vi "Radau5_Implicit RK Manager.vi"(9 "Jac Variant":variant, 10 "Jac Refnum":refnum<vi>, 11 "Simulation Data In":T1 {"Absolute tolerance" format="%.1e"; "Relative tolerance" format="%.1e"; "Output of T" format="%.1e"; "proposed step size" format="%.1e"; "min step size" format="%.1e"; "max step size" format="%.1e"; "final time" format="%.1e"; "step size" format="%.1e"; "initial time" format="%.1e"}) -> (3 "Simulation Data Out":T1 {"Absolute tolerance" format="%.1e"; "Relative tolerance" format="%.1e"; "Output of T" format="%.1e"; "proposed step size" format="%.1e"; "min step size" format="%.1e"; "max step size" format="%.1e"; "final time" format="%.1e"; "step size" format="%.1e"; "initial time" format="%.1e"})   [LabVIEW 2017, in "NI_DAE.lvlib"]
uses:
  <vilib>/gmath/NI_DAE.lvlib
  <vilib>/gmath/dae.llb/Radau5_Simulation Data.ctl
  <vilib>/gmath/dae.llb/Radau5_Diag Eval Stage.ctl
  <vilib>/gmath/dae.llb/Radau5_RK Status.ctl
  <vilib>/Analysis/baseanly.llb/A x Vector (Optimized).vi
  <vilib>/gmath/NI_Gmath.lvlib
  <vilib>/Analysis/NI_AALBase.lvlib
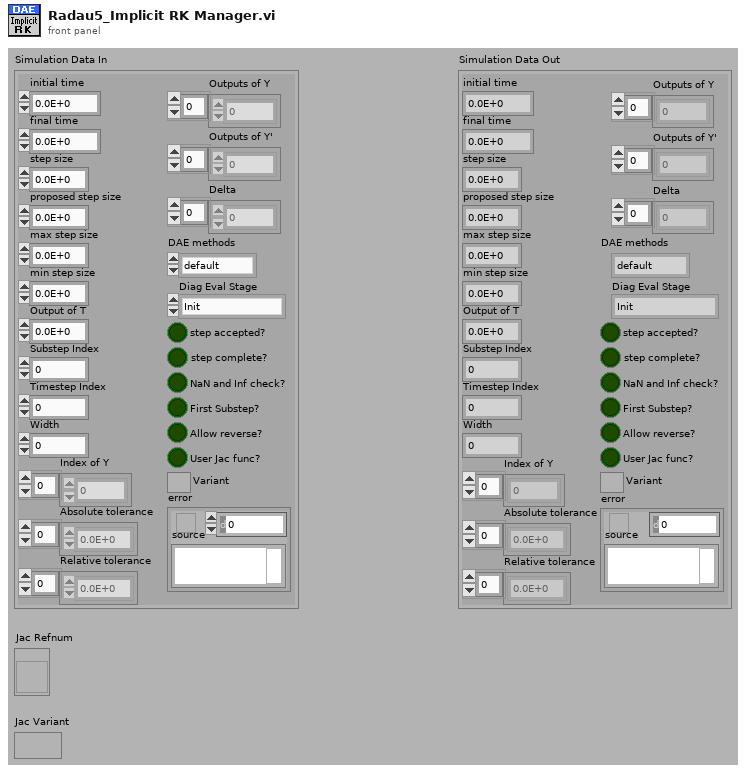
[diagram p1: front panel]
types:
  T1 = typedef "NI_DAE.lvlib/Radau5_Simulation Data.ctl" = cluster{"initial time":dbl, "final time":dbl, "step size":dbl, "proposed step size":dbl, "max step size":dbl, "min step size":dbl, "Output of T":dbl, "Substep Index":i32, "Timestep Index":i32, "Width":i32, "Absolute tolerance":dbl[], "Relative tolerance":dbl[], "Outputs of Y":dbl[], "Outputs of Y'":dbl[], "Delta":dbl[], "DAE methods":enum16{"default", "Radau IIA"}, "Diag Eval Stage":T2, "step accepted?":bool, "step complete?":bool, "NaN and Inf check?":bool, "First Substep?":bool, "Allow reverse?":bool, "error":errorcluster, "User Jac func?":bool, "Variant":variant, "Index of Y":i8[]}
  T2 = typedef "NI_DAE.lvlib/Radau5_Diag Eval Stage.ctl" = enum16{"Init", "Running", "Final", "End"}
  T3 = typedef "NI_DAE.lvlib/Radau5_RK Status.ctl" = enum16{"Init", "Predict", "Jacobian", "Newton", "error eval y y'", "error eval calc", "next step updata", "reset RK"}
  T4 = typedef "NI_DAE.lvlib/Radau5_Implicit RK Data.ctl" = cluster{"time":dbl, "Old time":dbl, "Step size":dbl, "Old step size":dbl, "Width":i32, "Newton index":i32, "Old Y(k)":dbl[], "Old Y'":dbl[], "Stage time":dbl[], "Old stage time":dbl[], "Increment Z":dbl[], "Delta Z":dbl[], "U":dbl[], "Old Delta Z":dbl[], "Y(k)":dbl[], "Y'":dbl[], "ErrorTolerance":dbl[], "Local error k+1":dbl[], "Old Local error k":dbl[], "Stage value of Y":dbl[][], "Stage value of Y'":dbl[][], "Old Stage value of Y":dbl[][], "Old Stage value of Y'":dbl[][], "RK status":T3, "do Jac?":bool, "Old Jac?":bool, "Do Newton?":bool, "Matrix J":T5, "Matrix M":T5, "Inverse of JM_1 matrix ":T5, "Inverse of JM_2 matrix":T6}
  T5 = typedef "NI_Matrix.lvlib/RealMatrix.ctl" = dbl[][]
  T6 = typedef "NI_Matrix.lvlib/ComplexMatrix.ctl" = cdb[][]
  T7 = typedef "NI_DAE.lvlib/Radau5_Newton Status.ctl" = enum16{"success", "unsuccess(iteration diverge)", "unsuccess(exceed max_N)", "unsuccess(conv rate too slow)", "Continue next Newton"}
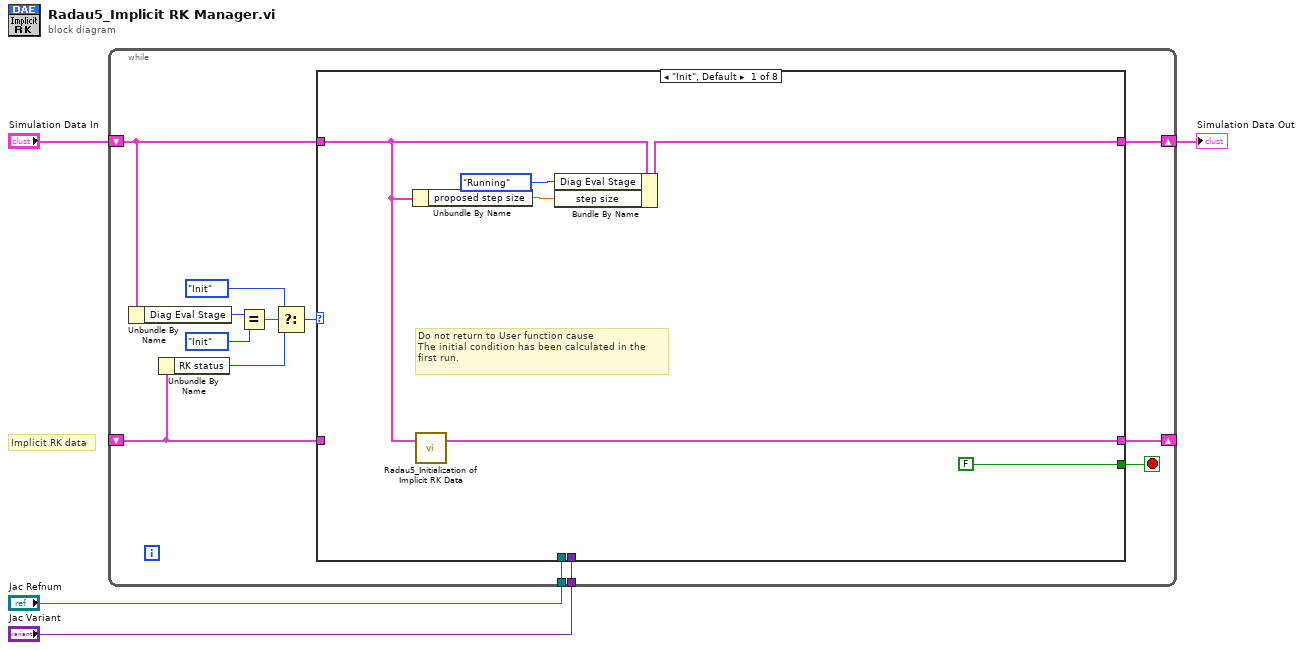
[diagram p0: block diagram]
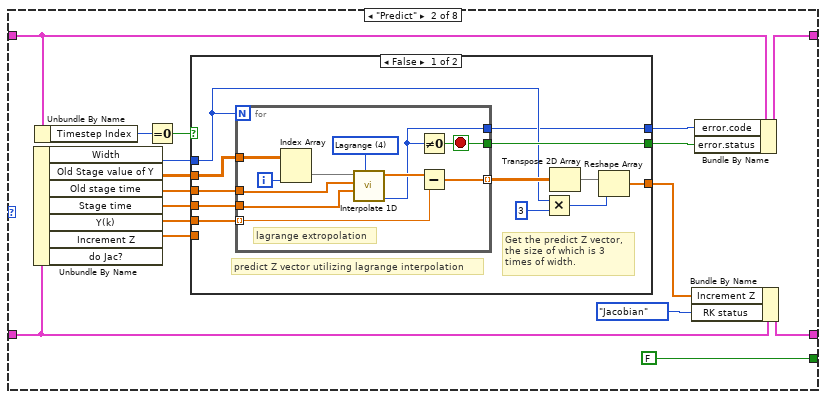
[diagram p2: hidden frame]
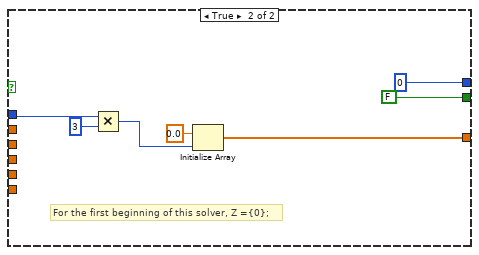
[diagram p3: hidden frame]
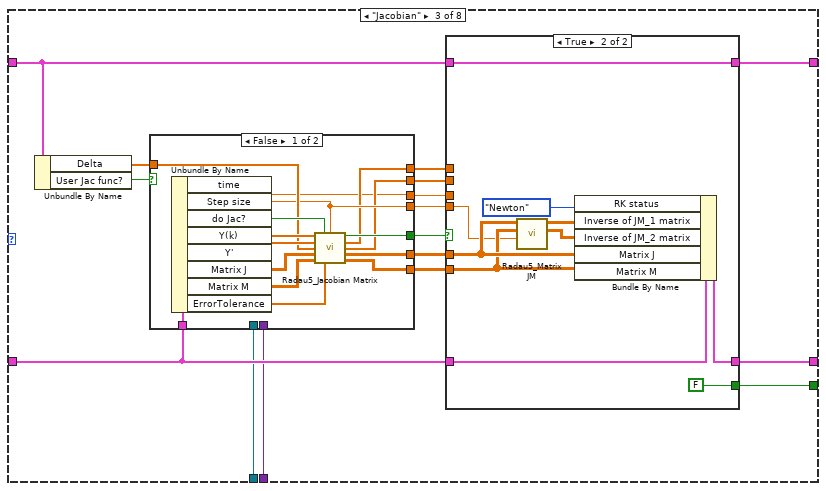
[diagram p4: hidden frame]
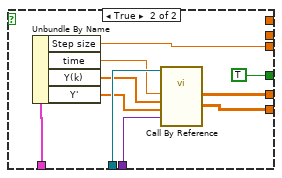
[diagram p5: hidden frame]
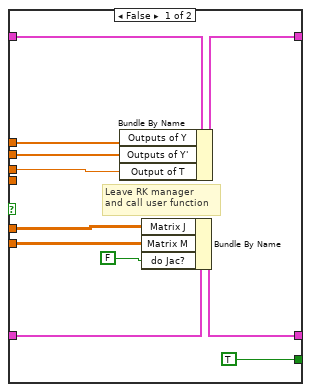
[diagram p6: hidden frame]
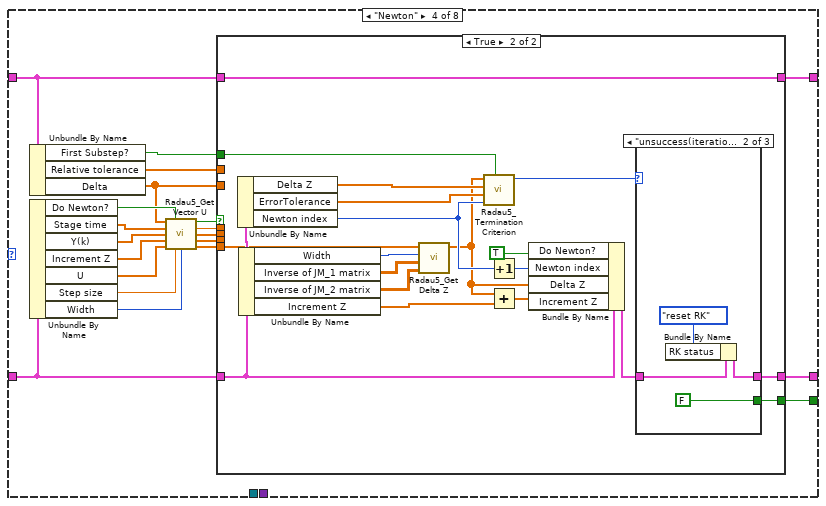
[diagram p7: hidden frame]
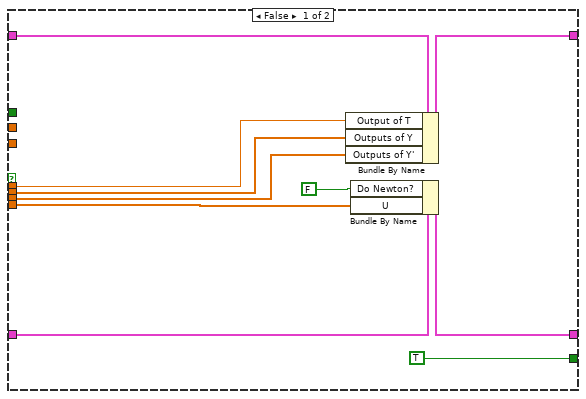
[diagram p8: hidden frame]
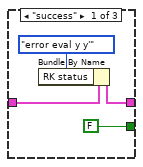
[diagram p9: hidden frame]
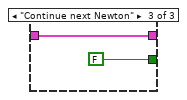
[diagram p10: hidden frame]
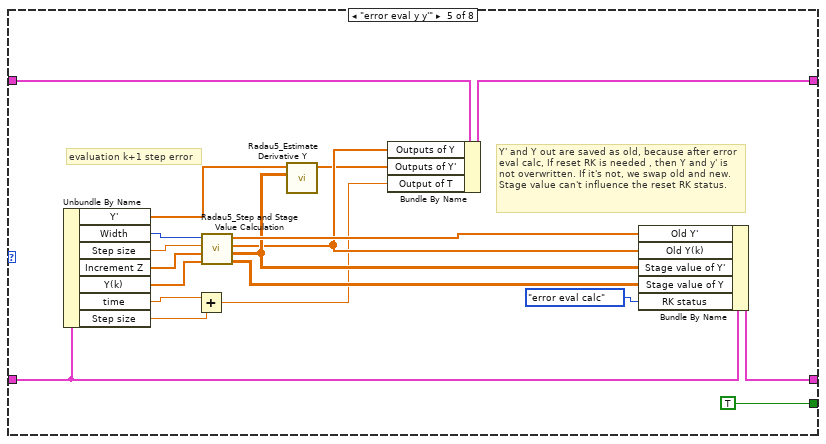
[diagram p11: hidden frame]
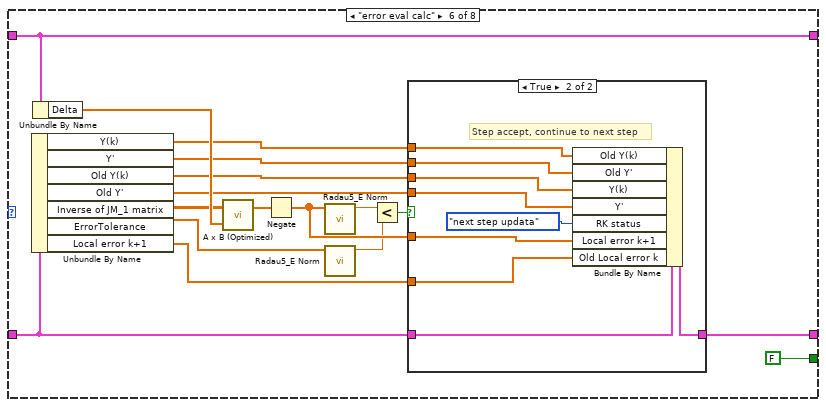
[diagram p12: hidden frame]
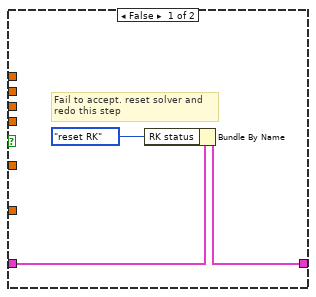
[diagram p13: hidden frame]
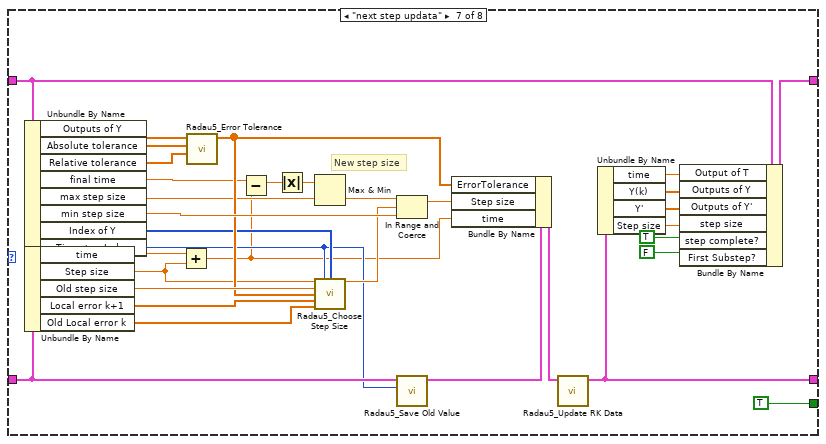
[diagram p14: hidden frame]
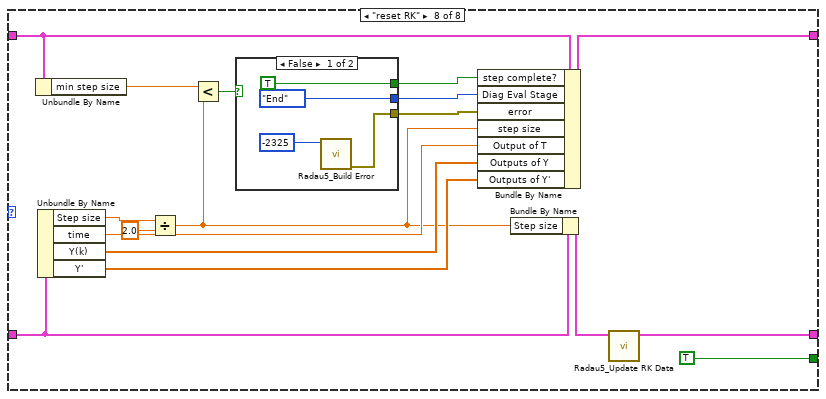
[diagram p15: hidden frame]
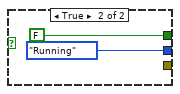
[diagram p16: hidden frame]
diagram:
  # "Implicit RK data"
  n1 = while {
    shift-right: [w7] -> _
    shift-left: _ -> [w8]
    shift-right: [w9] -> w3
    shift-left: "Simulation Data In" -> [w10]
    tunnel: "Jac Refnum" -> [w6]
    tunnel: "Jac Variant" -> [w5]
    stop <- w17 stop-if-true
    n2 = Unbundle By Name(w10) -> ("Diag Eval Stage"=w16:T2)
    n3 = Unbundle By Name(w8) -> ("RK status"=w12:T3)
    n4 = Equal?(x=w16, y=Radau5_Diag_Eval_Stage."Init") -> (x = y?=w14:bool)
    n5 = Select(t=Radau5_RK_Status."Init" ("RK status"), s=w14, f=w12) -> (s? t:f=w11:T3)
    n6 = case shown="\"Init\", Default" w11 {
      tunnel: w8 -> [_ w29 w84 w146 w207 w226 w266 w275]
      tunnel: [w22 w39 w81 w144 w205 w224 w260 w276] -> w7
      tunnel: [FALSE FALSE w79 w142 TRUE ("Newton flag") FALSE ("Newton flag") TRUE ("Newton flag") TRUE ("Newton flag")] -> w17
      tunnel: w10 -> [w19 w38 w78 w145 w210 w223 w262 w287]
      tunnel: [w20 w37 w75 w141 w209 w223 w261 w278] -> w9
      tunnel: w6 -> [_ _ w73 _ _ _ _ _]
      tunnel: w5 -> [_ _ w71 _ _ _ _ _]
      frame "Init", Default {
        # "Do not return to User function cause\nThe initial condition has been calculated in the \nfirst run."
        n7 = Unbundle By Name(w19) -> ("proposed step size"=w18:dbl)
        n8 = call <vilib>:"Radau5_Initialization of Implicit RK Data.vi"("Simulation Data"=w19) -> ("Implicit RK Data"=w22:T4)  [unwired: 2 in]
        n9 = Bundle By Name(cluster=w19, "Diag Eval Stage"=Radau5_Diag_Eval_Stage."Running", "step size"=w18) -> (w20:T1)
      }
      frame "Predict" {
        n10 = Unbundle By Name(w29) -> ("Width"=w34:i32, "Old Stage value of Y"=w33:dbl[][], "Old stage time"=w32:dbl[], "Stage time"=w31:dbl[], "Y(k)"=w30:dbl[], "Increment Z"=w28:dbl[])  [unwired: 1 out]
        n11 = Unbundle By Name(w38) -> ("Timestep Index"=w25:i32)
        n12 = Equal To 0?(x=w25) -> (x = 0?=w26:bool)
        n13 = case shown="False" w26 {
          tunnel: [w48 FALSE] -> w36
          tunnel: [w41 0 ("error")] -> w35
          tunnel: w34 -> [w47 w66]
          tunnel: w33 -> [w46 _]
          tunnel: w32 -> [w45 _]
          tunnel: w31 -> [w44 _]
          tunnel: w30 -> [w43 _]
          tunnel: [w42 w67] -> w27
          tunnel: w28 -> [_ _]
          frame False {
            # "Get the predict Z vector, \nthe size of which is 3 times of width."
            # "predict Z vector utilizing lagrange interpolation"
            n14 = for {
              N: w47 -> [_]
              tunnel: w45 -> [w59]
              tunnel: w46 -> [w62]
              tunnel: w44 -> [w58]
              tunnel: w43 -> [w56] mode=indexing
              tunnel: [w55] -> w52 mode=indexing
              tunnel: [w54] -> w48
              tunnel: [w53] -> w41
              i -> [w61]
              stop <- w54 stop-if-true
              w63 = 4 items=["nearest", "linear", "spline", "cubic Hermite", "Lagrange"] ("method")
              # "lagrange extropolation"
              n15 = Index Array(array=w62, index (col)=w61) -> (element=w60:dbl[])  [unwired: 1 in]
              n16 = call <vilib>:"Interpolate 1D.vi"("method"=w63, "xi"=w58, "X"=w59, "Y"=w60) -> ("error"=w53:i32, "yi"=w57:dbl[])  [unwired: 2 in, 4 out]
              n17 = Not Equal To 0?(x=w53) -> (x != 0?=w54:bool)
              n18 = Subtract(x=w57, y=w56) -> (x-y=w55:dbl[])
            }
            n19 = Multiply(x=w47, y=3 ("x")) -> (x*y=w49:i32)
            n20 = Transpose 2D Array(2D array=w52) -> (transposed array=w51:dbl[][])
            n21 = Reshape Array(w51, w49) -> (w42:dbl[])
          }
          frame True {
            # "For the first beginning of this solver, Z ={0};"
            n22 = Multiply(x=w66, y=3) -> (x*y=w64:i32)
            n23 = Initialize Array(0.0 ("element"), w64) -> (w67:dbl[])
          }
        }
        n24 = Bundle By Name(cluster=w29, "Increment Z"=w27, "RK status"=Radau5_RK_Status."Jacobian") -> (w39:T4)
        n25 = Bundle By Name(cluster=w38, "error.code"=w35, "error.status"=w36) -> (w37:T1)
      }
      frame "Jacobian" {
        n26 = Unbundle By Name(w78) -> ("Delta"=w86:dbl[], "User Jac func?"=w72:bool)
        n27 = case shown="False" w72 {
          tunnel: w86 -> [w95 _]
          tunnel: [w94 TRUE ("Ready")] -> w85
          tunnel: w84 -> [w93 w111]
          tunnel: [w92 w106] -> w83
          tunnel: [w91 w105] -> w82
          tunnel: [w90 w103] -> w80
          tunnel: [w89 _] -> w77
          tunnel: [w88 _] -> w76
          tunnel: [w87 _] -> w74
          tunnel: w73 -> [_ w110]
          tunnel: w71 -> [_ w102]
          frame False {
            n28 = Unbundle By Name(w93) -> ("time"=w87:dbl, "Step size"=w90:dbl, "do Jac?"=w96:bool, "Y(k)"=w97:dbl[], "Y'"=w98:dbl[], "Matrix J"=w101:T5, "Matrix M"=w100:T5, "ErrorTolerance"=w99:dbl[])
            n29 = call <vilib>:"Radau5_Jacobian Matrix.vi"("Y(k)"=w97, "do Jac?"=w96, "Step size"=w90, "Y'"=w98, "Fout"=w95, "Matrix J"=w101, "Matrix M"=w100, "ErrorTolerance"=w99) -> ("Ready"=w94:bool, "Y(k)"=w89:dbl[], "Y'"=w88:dbl[], "Matrix J"=w92:T5, "Matrix M"=w91:T5)  [unwired: 3 in]
          }
          frame True {
            n30 = Unbundle By Name(w111) -> ("Step size"=w103:dbl, "time"=w109:dbl, "Y(k)"=w108:dbl[], "Y'"=w107:dbl[])
            n31 = call-by-ref "?"(reference=w110, "Variant"=w102, "Y'"=w107, "Y"=w108, "Time"=w109) -> ("Real Matrix 2"=w105:T5, "Real Matrix"=w106:T5)  [unwired: 1 in, 3 out]
          }
        }
        n32 = case shown="True" w85 {
          tunnel: w84 -> [w121 w132]
          tunnel: w83 -> [w120 w130]
          tunnel: w82 -> [w119 w129]
          tunnel: [w118 w131] -> w81
          tunnel: w80 -> [_ w126]
          tunnel: [TRUE FALSE] -> w79
          tunnel: w78 -> [w116 w124]
          tunnel: w77 -> [w115 _]
          tunnel: w76 -> [w114 _]
          tunnel: [w113 w124] -> w75
          tunnel: w74 -> [w112 _]
          frame False {
            # "Leave RK manager\nand call user function"
            n33 = Bundle By Name(cluster=w116, "Outputs of Y"=w115, "Outputs of Y'"=w114, "Output of T"=w112) -> (w113:T1)
            n34 = Bundle By Name(cluster=w121, "Matrix J"=w120, "Matrix M"=w119, "do Jac?"=FALSE) -> (w118:T4)
          }
          frame True {
            n35 = call <vilib>:"Radau5_Matrix JM.vi"("Step size"=w126, "Matrix M"=w129, "Matrix J"=w130) -> ("Inverse of Matrix JM_2"=w127:T6, "Inverse of Matrix JM_1"=w128:T5)  [unwired: 7 in]
            n36 = Bundle By Name(cluster=w132, "RK status"=Radau5_RK_Status."Newton", "Inverse of JM_1 matrix"=w128, "Inverse of JM_2 matrix"=w127, "Matrix J"=w130, "Matrix M"=w129) -> (w131:T4)
          }
        }
      }
      frame "Newton" {
        n37 = Unbundle By Name(w145) -> ("First Substep?"=w134:bool, "Relative tolerance"=w143:dbl[], "Delta"=w135:dbl[])
        n38 = Unbundle By Name(w146) -> ("Do Newton?"=w139:bool, "Stage time"=w136:dbl[], "Y(k)"=w137:dbl[], "Increment Z"=w138:dbl[], "U"=w152:dbl[], "Step size"=w133:dbl, "Width"=w140:i32)
        n39 = call <vilib>:"Radau5_Get Vector U.vi"("Delta In"=w135, "Flag"=w139, "Stage time"=w136, "Step Value Y"=w137, "Vector Z in"=w138, "Vector U in"=w152, "Step size"=w133, "Width"=w140) -> ("Vector U Ready?"=w151:bool, "Stage time out"=w150:dbl, "Stage Y out"=w149:dbl[], "Stage Y' out"=w148:dbl[], "Vector U out"=w147:dbl[])  [unwired: 3 in]
        n40 = case shown="True" w151 {
          tunnel: w150 -> [w160 _]
          tunnel: w149 -> [w155 _]
          tunnel: w148 -> [w154 _]
          tunnel: w147 -> [w156 w171]
          tunnel: w146 -> [w157 w178]
          tunnel: w145 -> [w161 w165]
          tunnel: [w158 w168] -> w144
          tunnel: w135 -> [_ _]
          tunnel: w143 -> [_ _]
          tunnel: [TRUE ("Newton flag") w175] -> w142
          tunnel: [w159 w165] -> w141
          tunnel: w134 -> [_ w167]
          frame False {
            n41 = Bundle By Name(cluster=w161, "Output of T"=w160, "Outputs of Y"=w155, "Outputs of Y'"=w154) -> (w159:T1)
            n42 = Bundle By Name(cluster=w157, "Do Newton?"=FALSE, "U"=w156) -> (w158:T4)
          }
          frame True {
            n43 = Unbundle By Name(w178) -> ("Delta Z"=w164:dbl[], "ErrorTolerance"=w169:dbl[], "Newton index"=w166:i32)
            n44 = Unbundle By Name(w178) -> ("Width"=w172:i32, "Inverse of JM_1 matrix"=w181:T5, "Inverse of JM_2 matrix"=w180:T6, "Increment Z"=w170:dbl[])
            n45 = call <vilib>:"Radau5_Get Delta Z.vi"("Inverse Matrix JM_2"=w180, "Inverse Matrix JM_1"=w181, "Width"=w172, "Vector U in"=w171) -> ("Delta Z out"=w163:dbl[])  [unwired: 7 in]
            n46 = call <vilib>:"Radau5_Termination Criterion.vi"("First call?"=w167, "Newton index"=w166, "Error TOL"=w169, "Old Delta Z"=w164, "Delta Z"=w163) -> ("Newton status"=w177:T7)  [unwired: 6 in]
            n47 = Increment(x=w166) -> (x+1=w174:i32)
            n48 = Add(x=w163, y=w170) -> (x+y=w179:dbl[])
            n49 = Bundle By Name(cluster=w178, "Do Newton?"=TRUE, "Newton index"=w174, "Delta Z"=w163, "Increment Z"=w179) -> (w176:T4)
            n50 = case shown="\"unsuccess(iteration diverge)\", Default" w177 {
              tunnel: w176 -> [w185 w188 w191]
              tunnel: [w183 w187 w191] -> w168
              tunnel: [FALSE ("Newton flag") FALSE ("Newton flag") FALSE ("Newton flag")] -> w175
              frame "success" {
                n51 = Bundle By Name(cluster=w185, "RK status"=Radau5_RK_Status."error eval y y'") -> (w183:T4)
              }
              frame "unsuccess(iteration diverge)", Default {
                n52 = Bundle By Name(cluster=w188, "RK status"=Radau5_RK_Status."reset RK") -> (w187:T4)
              }
              frame "Continue next Newton" {
              }
            }
          }
        }
      }
      frame "error eval y y'" {
        # "Y' and Y out are saved as old, because after error eval calc, If reset RK is needed , then Y and y' is not overwritten. If it's not, we swap old and new.\nStage value can't influence the reset RK status."
        # "evaluation k+1 step error"
        n53 = Unbundle By Name(w207) -> ("Y'"=w194:dbl[], "Width"=w204:i32, "Step size"=w192:dbl, "Increment Z"=w203:dbl[], "Y(k)"=w202:dbl[], "time"=w196:dbl, "Step size"=w197:dbl)
        n54 = Add(x=w196, y=w197) -> (x+y=w195:dbl)
        n55 = call <vilib>:"Radau5_Step and Stage Value Calculation.vi"("Y(k)"=w202, "Increment Z"=w203, "Step size"=w192, "Width"=w204) -> ("Stage value of Y"=w200:dbl[][], "Stage value of Y'"=w199:dbl[][], "Y(k+1) out"=w198:dbl[], "Y'(k+1) out"=w201:dbl[])  [unwired: 4 in]
        n56 = call <vilib>:"Radau5_Estimate Derivative Y.vi"("Stage Y'"=w199, "Old Y'"=w194) -> ("Estimate Y' out"=w193:dbl[])  [unwired: 9 in]
        n57 = Bundle By Name(cluster=w210, "Outputs of Y"=w198, "Outputs of Y'"=w193, "Output of T"=w195) -> (w209:T1)
        n58 = Bundle By Name(cluster=w207, "Old Y'"=w201, "Old Y(k)"=w198, "Stage value of Y'"=w199, "Stage value of Y"=w200, "RK status"=Radau5_RK_Status."error eval calc") -> (w205:T4)
      }
      frame "error eval calc" {
        n59 = Unbundle By Name(w226) -> ("Y(k)"=w219:dbl[], "Y'"=w218:dbl[], "Old Y(k)"=w217:dbl[], "Old Y'"=w216:dbl[], "Inverse of JM_1 matrix"=w220:T5, "ErrorTolerance"=w215:dbl[], "Local error k+1"=w225:dbl[])
        n60 = Unbundle By Name(w223) -> ("Delta"=w227:dbl[])
        n61 = call-poly <vilib>:"A x B (Optimized).vi"("Vector"=w227, "A"=w220) -> ("A x Vector"=w221:dbl[])  [unwired: 1 out]
        n62 = Negate(x=w221) -> (-x=w214:dbl[])
        n63 = call <vilib>:"Radau5_E Norm.vi"("Vector in"=w214) -> ("Norm output"=w213:dbl)  [unwired: 10 in]
        n64 = call <vilib>:"Radau5_E Norm.vi"("Vector in"=w215) -> ("Norm output"=w212:dbl)  [unwired: 10 in]
        n65 = Less?(x=w213, y=w212) -> (x < y?=w211:bool)
        n66 = case shown="True" w211 {
          tunnel: w226 -> [w230 w239]
          tunnel: w225 -> [_ w238]
          tunnel: [w228 w237] -> w224
          tunnel: w214 -> [_ w235]
          tunnel: w219 -> [_ w232]
          tunnel: w218 -> [_ w233]
          tunnel: w217 -> [_ w231]
          tunnel: w216 -> [_ w234]
          frame False {
            # "Fail to accept. reset solver and redo this step"
            n67 = Bundle By Name(cluster=w230, "RK status"=Radau5_RK_Status."reset RK") -> (w228:T4)
          }
          frame True {
            # "Step accept, continue to next step"
            n68 = Bundle By Name(cluster=w239, "Old Y(k)"=w232, "Old Y'"=w233, "Y(k)"=w231, "Y'"=w234, "RK status"=Radau5_RK_Status."next step updata", "Local error k+1"=w235, "Old Local error k"=w238) -> (w237:T4)
          }
        }
      }
      frame "next step updata" {
        # "New step size"
        n69 = Unbundle By Name(w262) -> ("Outputs of Y"=w271:dbl[], "Absolute tolerance"=w270:dbl[], "Relative tolerance"=w269:dbl[], "final time"=w249:dbl, "max step size"=w246:dbl, "min step size"=w255:dbl, "Index of Y"=w250:i8[], "Timestep Index"=w243:i32)
        n70 = Unbundle By Name(w266) -> ("time"=w241:dbl, "Step size"=w242:dbl, "Old step size"=w272:dbl, "Local error k+1"=w268:dbl[], "Old Local error k"=w267:dbl[])
        n71 = Add(x=w241, y=w242) -> (x+y=w240:dbl)
        n72 = call <vilib>:"Radau5_Error Tolerance.vi"("Relative Tolerance"=w269, "Absolute Tolerance"=w270, "Y in"=w271) -> ("Error tolerance"=w253:dbl[])  [unwired: 8 in]
        n73 = Subtract(x=w249, y=w240) -> (x-y=w248:dbl)
        n74 = Absolute Value(x=w248) -> (abs(x)=w247:dbl)
        n75 = Max & Min(x=w247, y=w246) -> (min(x,y)=w245:dbl)  [unwired: 1 out]
        n76 = call <vilib>:"Radau5_Choose Step Size.vi"("step size"=w242, "Step index"=w243, "Index of Y"=w250, "old step size"=w272, "ErrorTolerance"=w253, "Local error"=w268, "Old Local error"=w267) -> ("New step size"=w244:dbl)  [unwired: 8 in]
        n77 = In Range and Coerce(upper limit=w245, x=w244, lower limit=w255) -> (coerced(x)=w254:dbl)  [unwired: 1 out]
        n78 = call <vilib>:"Radau5_Save Old Value.vi"("Timestep index"=w243, "Implicit RK Data In"=w266) -> ("Implicit RK Data Out"=w265:T4)  [unwired: 9 in]
        n79 = Bundle By Name(cluster=w265, "ErrorTolerance"=w253, "Step size"=w254, "time"=w240) -> (w264:T4)
        n80 = call <vilib>:"Radau5_Update RK Data.vi"("Implicit RK Data In"=w264) -> ("Implicit RK Data Out"=w260:T4)  [unwired: 10 in]
        n81 = Unbundle By Name(w260) -> ("time"=w259:dbl, "Y(k)"=w258:dbl[], "Y'"=w257:dbl[], "Step size"=w251:dbl)
        n82 = Bundle By Name(cluster=w262, "Output of T"=w259, "Outputs of Y"=w258, "Outputs of Y'"=w257, "step size"=w251, "step complete?"=TRUE, "First Substep?"=FALSE) -> (w261:T1)
      }
      frame "reset RK" {
        n83 = Unbundle By Name(w287) -> ("min step size"=w286:dbl)
        n84 = Unbundle By Name(w275) -> ("Step size"=w274:dbl, "time"=w282:dbl, "Y(k)"=w281:dbl[], "Y'"=w280:dbl[])
        n85 = Divide(x=w274, y=2.0) -> (x/y=w273:dbl)
        n86 = Less?(x=w286, y=w273) -> (x < y?=w285:bool)
        n87 = case shown="False" w285 {
          tunnel: [Radau5_Diag_Eval_Stage."End" ("Diag Eval Stage") Radau5_Diag_Eval_Stage."Running" ("Diag Eval Stage")] -> w284
          tunnel: [w291 _] -> w283
          tunnel: [TRUE ("step complete?") FALSE ("step complete?")] -> w279
          frame False {
            n88 = call <vilib>:"Radau5_Build Error.vi"("error code"=-2325) -> ("error out"=w291:errorcluster)  [unwired: 10 in]
          }
          frame True {
          }
        }
        n89 = Bundle By Name(cluster=w287, "step complete?"=w279, "Diag Eval Stage"=w284, "error"=w283, "step size"=w273, "Output of T"=w282, "Outputs of Y"=w281, "Outputs of Y'"=w280) -> (w278:T1)
        n90 = Bundle By Name(cluster=w275, "Step size"=w273) -> (w277:T4)
        n91 = call <vilib>:"Radau5_Update RK Data.vi"("Implicit RK Data In"=w277) -> ("Implicit RK Data Out"=w276:T4)  [unwired: 10 in]
      }
    }
  }
  "Simulation Data Out" <- w3
